vi "Measurement Logic.vi"(8 "error in":errorcluster, 9 "measurement configuration":T2 {"Baudrate" format="%x"; "FD Baudrate" format="%x"}, 10 "measure call context in":refnum<class "Measure Call Context.lvclass">, 11 "Stop OOB Server UE":refnum<user-event>) -> (0 "error out":errorcluster, 1 "measurement results":T1, 2 "measure call context out":refnum<class "Measure Call Context.lvclass">)   [LabVIEW 2025, in "CAN-LIN Raw Bus Capture.lvclass"]
doc: "Contains the core logic for executing the measurement."
uses:
  CAN-LIN Raw Bus Capture.lvclass
  <vilib>/Plug-In SDKs/Measurements/Measure Call Context/Measure Call Context.lvclass
  Measurement Configuration.ctl
  CAN-LIN Raw Bus Capture UI/Toggle.ctl
  Measurement Results.ctl
  <vilib>/xnet/xnet.llb/XNET Read (State LIN Comm).vi
  CAN-LIN Raw Bus Capture.lvclass/CAN-LIN Raw Bus Capture.ctl
  <vilib>/xnet/xnet.llb/XNET Read (State CAN Comm).vi
  <vilib>/xnet/xnet.llb/XNET Read (Frame CAN).vi
  <vilib>/xnet/xnet.llb/XNET Read (Frame LIN).vi
  OOB Data Transfer/OOB Data Transfer.lvlib
  session-management/xnetCAN/Session Management xnetCAN.lvlib
  <vilib>/Plug-In SDKs/Clients/Session Management V1/Session Reservation/Session Reservation.lvclass
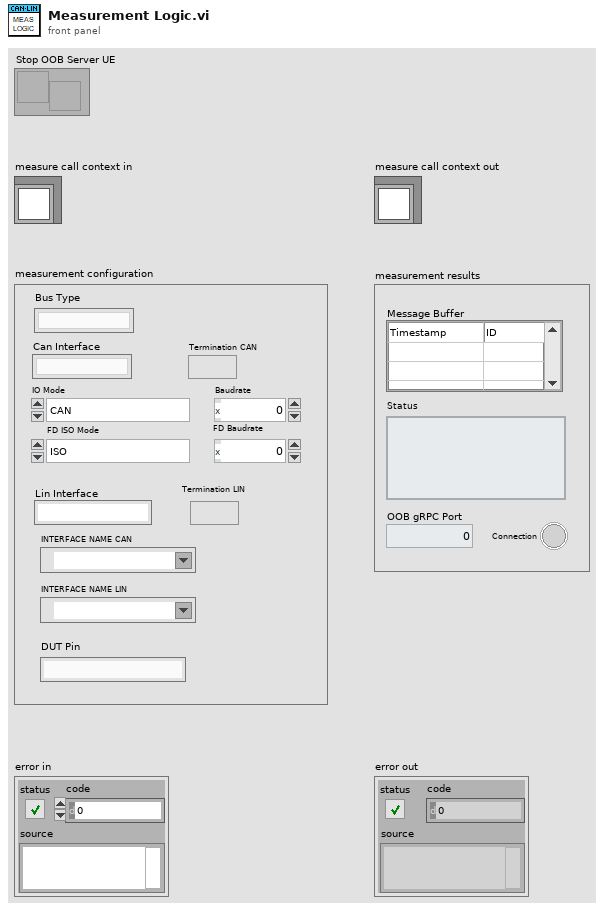
[diagram p1: front panel]
types:
  T1 = typedef "CAN-LIN Raw Bus Capture.lvclass/Measurement Results.ctl" = cluster{"Message Buffer":string[][], "Status":string, "OOB gRPC Port":i32, "Connection":bool}
  T2 = typedef "CAN-LIN Raw Bus Capture.lvclass/Measurement Configuration.ctl" = cluster{"Termination CAN":T3, "FD Baudrate":u32, "Baudrate":u32, "FD ISO Mode":enum32{"ISO", "Legacy ISO", "Non-ISO"}, "IO Mode":enum32{"CAN", "CAN FD", "CAN FD + BRS"}, "Termination LIN":T3, "Can Interface":string, "Lin Interface":string, "Bus Type":string, "INTERFACE NAME CAN":refnum<k21>, "INTERFACE NAME LIN":refnum<k21>, "DUT Pin":string}
  T3 = typedef "Toggle.ctl" = bool
  T4 = typedef "Session Management xnetCAN.lvlib/Connection with Session.ctl" = cluster{"connection":T5, "session":string}
  T5 = typedef "NI Session Management V1 Client.lvlib/Session Reservation.lvclass/Connection.ctl" = cluster{"pin or relay name":string, "site":i32, "instrument type id":string, "channel":string}
  T6 = typedef "OOB Data Transfer.lvlib/OOB to Logic Data.ctl" = cluster{"PauseResume":bool, "Export":string, "STOP":bool}
  T7 = typedef "XNET Frame CAN.ctl" = cluster{"timestamp":timestamp, "payload":u8[], "identifier":u32, "type":T8, "extended?":bool, "echo?":bool}
  T8 = typedef "XNET Frame Type CAN.ctl" = u8
  T9 = typedef "XNET CAN Comm.ctl" = cluster{"fault code":i32, "fault?":bool, "communication state":T10, "last error":T11, "receive error counter":u8, "transmit error counter":u8, "transceiver error?":bool, "sleep?":bool}
  T10 = typedef "XNET CAN Comm State.ctl" = u8
  T11 = typedef "XNET CAN Last Err.ctl" = u8
  T12 = typedef "XNET Frame LIN.ctl" = cluster{"timestamp":timestamp, "payload":u8[], "identifier":u32, "type":T13, "event ID":u8, "event slot?":bool, "echo?":bool}
  T13 = typedef "XNET Frame Type LIN.ctl" = u8
  T14 = typedef "XNET LIN Comm.ctl" = cluster{"fault code":i32, "fault?":bool, "communication state":T15, "last error":T16, "last error received":u8, "last error expected":u8, "last error identifier":u8, "sleep?":bool, "transceiver ready?":bool, "schedule index":u8}
  T15 = typedef "XNET LIN Comm State.ctl" = u8
  T16 = typedef "XNET LIN Last Err.ctl" = u8
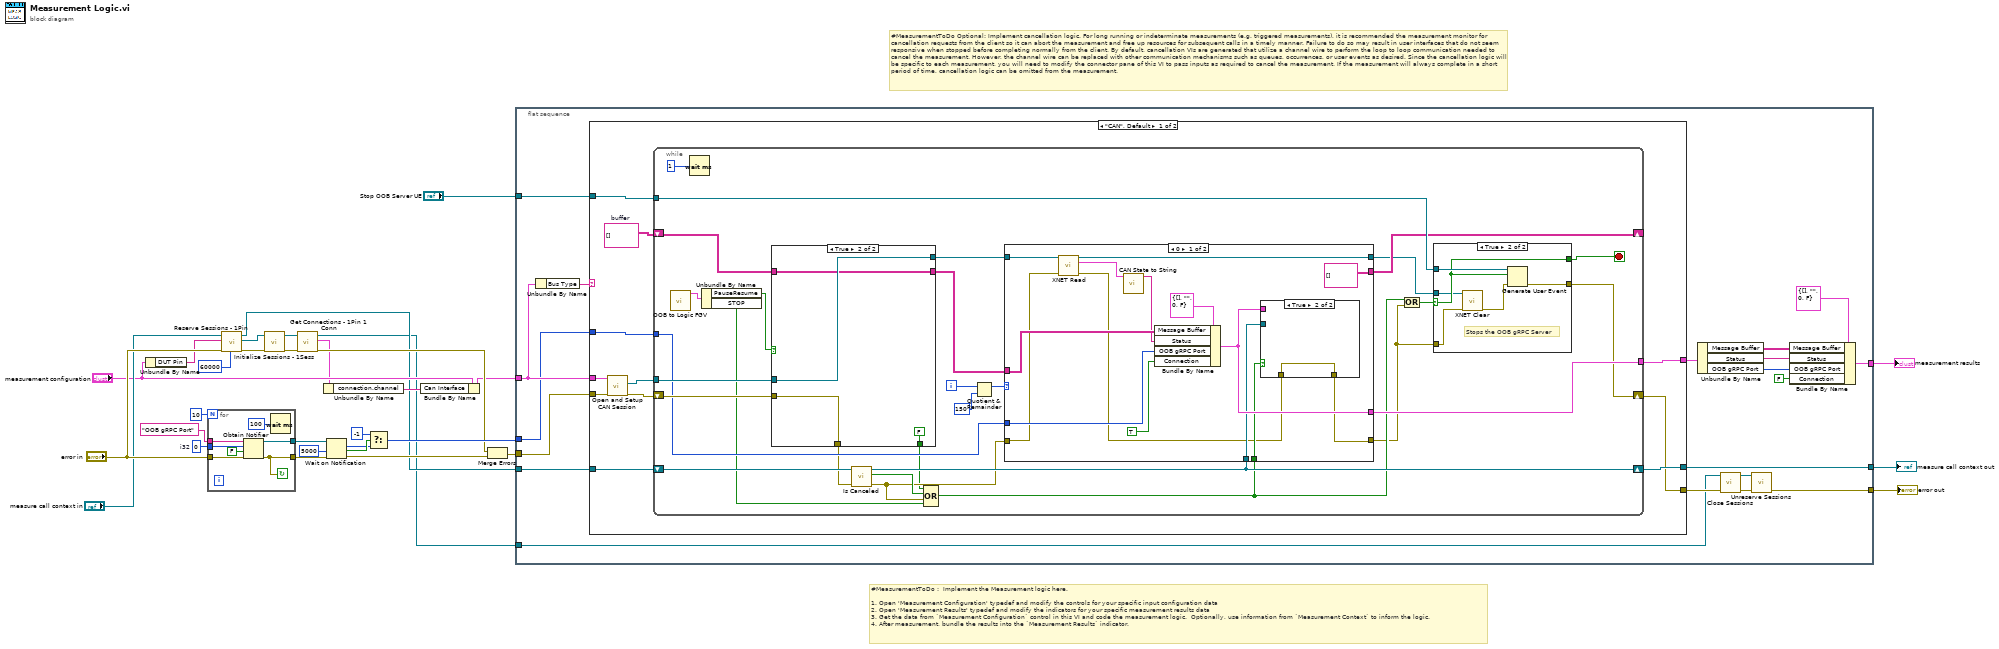
[diagram p0: block diagram]
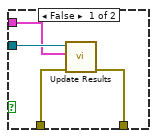
[diagram p2: hidden frame]
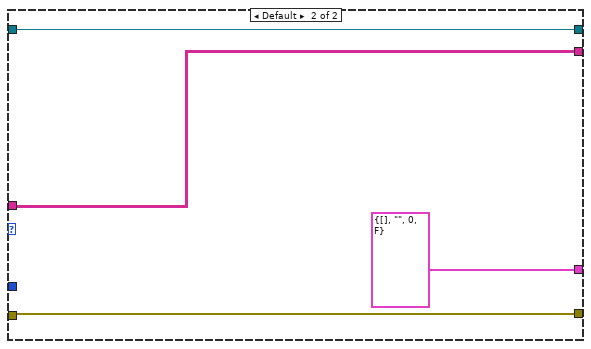
[diagram p3: hidden frame]
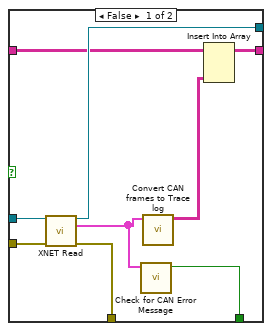
[diagram p4: hidden frame]
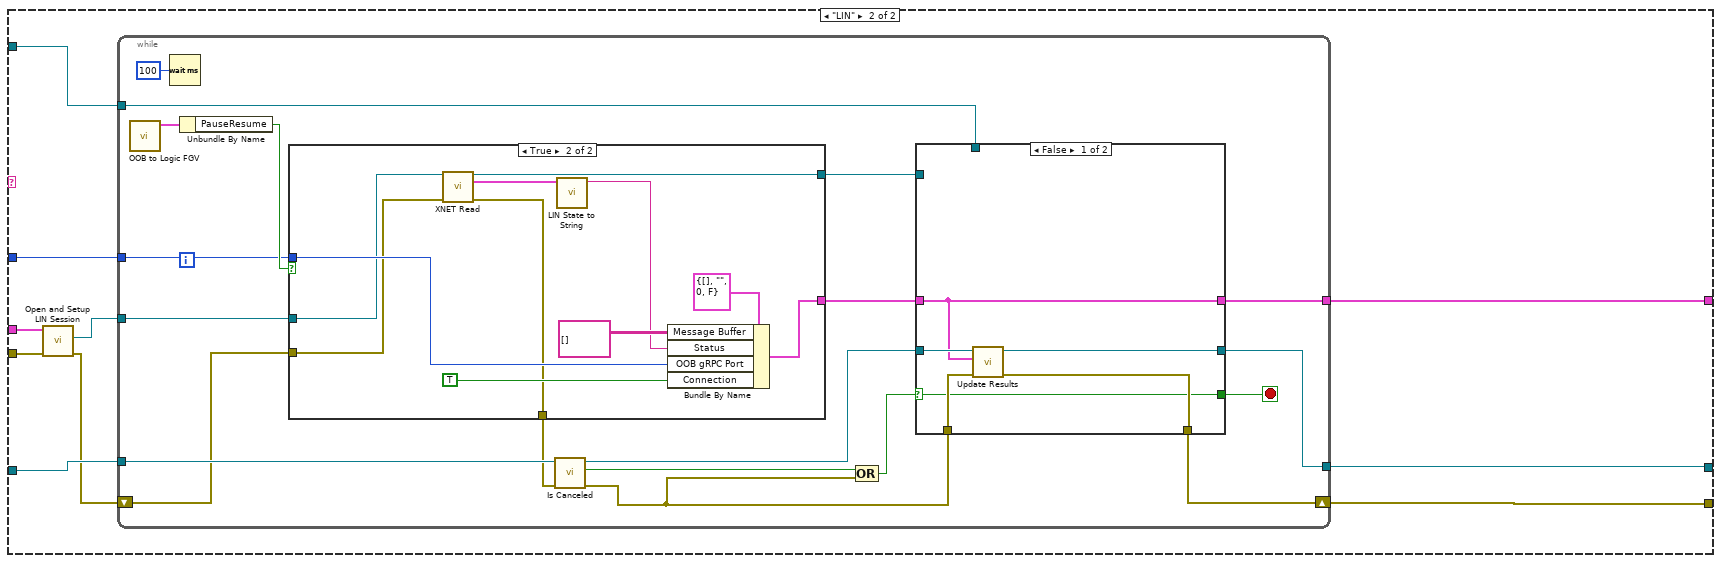
[diagram p6: hidden frame]
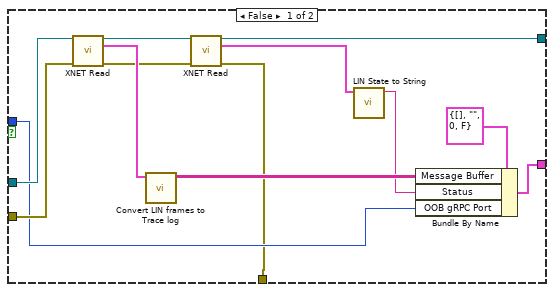
[diagram p7: hidden frame]
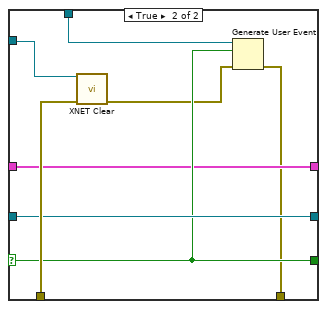
[diagram p8: hidden frame]
diagram:
  w23 = 0  # i32
  # "#MeasurementToDo Optional: Implement cancellation logic. For long running or indeterminate measurements (e.g. triggered measurements), it is recommended the measurement monitor for cancellation requests from the client so it can abort the measurement and free up resources for subsequent calls in a timely manner. Failure to do so may result in user interfaces that do not seem responsive when stopped before completing normally from the client. By default, cancellation VIs are generated that utilize a channel wire to perform the loop to loop communication needed to cancel the measurement. However, the channel wire can be replaced with other communication mechanisms such as queues, occurrences, or user events as desired. Since the cancellation logic will be specific to each measurement, you will need to modify the connector pane of this VI to pass inputs as required to cancel the measurement. If the measurement will always complete in a short period of time, cancellation logic can be omitted from the measurement."
  # "#MeasurementToDo :  Implement the Measurement logic here.\n\n1. Open 'Measurement Configuration' typedef and modify the controls for your specific input configuration data\n2. Open 'Measurement Results' typedef and modify the indicators for your specific measurement results data\n3. Get the data from `Measurement Configuration` control in this VI and code the measurement logic.  Optionally, use information from `Measurement Context` to inform the logic.\n4. After measurement, bundle the results into the `Measurement Results` indicator."
  n1 = Unbundle By Name("measurement configuration") -> ("DUT Pin"=w6:string)
  n2 = for {
    N: 10 -> [_]
    tunnel: [w35] -> w27
    tunnel: [w37] -> w26
    tunnel: "OOB gRPC Port" ("name (unnamed)") -> [w34]
    tunnel: w23 -> [w33]
    tunnel: "error in" -> [w32]
    stop <- w35 continue-if-true
    n3 = Obtain Notifier(name (unnamed)=w34, notification data type=w33, create if not found? (T)=FALSE, error in (no error)=w32) -> (notifier out=w37:refnum<notifier>, error out=w35:errorcluster)  [unwired: 1 out]
    n4 = Wait (ms)(milliseconds to wait=u32 100) -> ()  [unwired: 1 out]
  }
  n5 = call <vilib>:"Reserve Sessions - 1Pin.vi"("timeout (ms)"=60000 ("timeout in milliseconds"), "error in"="error in", "pin or relay name"=w6, "measurement context in"="measure call context in") -> ("error out"=w14:errorcluster, "session reservation out"=w15:refnum<class "Session Reservation.lvclass">, "measurement context out"=w2:refnum<class "Measure Call Context.lvclass">)  [unwired: 5 in]
  n6 = call "Initialize Sessions - 1Sess.vi"("error in"=w14, "session reservation in"=w15) -> ("error out"=w12:errorcluster, "session reservation out"=w13:refnum<class "Session Reservation.lvclass">)  [unwired: 6 in, 2 out]
  n7 = call "Get Connections - 1Pin 1 Conn.vi"("error in"=w12, "session reservation in"=w13) -> ("error out"=w9:errorcluster, "connection"=w4:T4, "session reservation out"=w1:refnum<class "Session Reservation.lvclass">)  [unwired: 7 in]
  n8 = Unbundle By Name(w4) -> ("connection.channel"=w3:string)
  n9 = Wait on Notification(notifier=w26, timeout in ms (-1)=5000, error in (no error)=w27) -> (notification=w20:i32, timed out?=w21:bool, error out=w18:errorcluster)  [unwired: 1 in, 1 out]
  n10 = Select(t=-1, s=w21, f=w20) -> (s? t:f=w17:i32)
  n11 = Bundle By Name(cluster="measurement configuration", "Can Interface"=w3) -> (w5:T2)
  n12 = Merge Errors(w9, w18) -> (w10:errorcluster)
  n13 = flat-sequence {
    tunnel: w5 -> [w56]
    tunnel: [w49] -> w31
    tunnel: w10 -> [w54]
    tunnel: w2 -> [w55]
    tunnel: [w41] -> w30
    tunnel: [w53] -> w29
    tunnel: "Stop OOB Server UE" -> [w52]
    tunnel: w17 -> [w51]
    tunnel: w1 -> [w40]
    frame #0 {
      n14 = Unbundle By Name(w56) -> ("Bus Type"=w57:string)
      n15 = case shown="\"CAN\", Default" w57 {
        tunnel: w56 -> [w66 w145]
        tunnel: w55 -> [w65 w148]
        tunnel: w54 -> [w64 w147]
        tunnel: [w63 w149] -> w50
        tunnel: [w62 w151] -> w53
        tunnel: [w61 w150] -> w42
        tunnel: w52 -> [w60 w143]
        tunnel: w51 -> [w59 w142]
        frame "CAN", Default {
          w58 = string[][] []  # buffer
          n16 = call "Open and Setup CAN Session.vi"("error in"=w64, "measurement configuration"=w66) -> ("error out"=w67:errorcluster, "session out"=w68:refnum<k21>)  [unwired: 8 in]
          n17 = while {
            tunnel: [w87] -> w63
            shift-right: [w76] -> w61
            shift-left: w67 -> [w94]
            tunnel: w68 -> [w93]
            tunnel: w60 -> [w92]
            tunnel: w59 -> [w89]
            shift-right: [w81] -> w62
            shift-left: w65 -> [w95]
            shift-right: [w78] -> _
            shift-left: w58 -> [w83]
            i -> [w86]
            stop <- w70 stop-if-true
            n18 = call "OOB to Logic FGV.vi"() -> ("OOB to Logic Data out"=w90:T6)  [unwired: 10 in, 1 out]
            n19 = Wait (ms)(milliseconds to wait=u32 1) -> ()  [unwired: 1 out]
            n20 = Unbundle By Name(w90) -> ("PauseResume"=w77:bool, "STOP"=w69:bool)
            n21 = case shown="True" w77 {
              tunnel: w94 -> [w129 w133]
              tunnel: [w128 w133] -> w88
              tunnel: [w127 w132] -> w79
              tunnel: w93 -> [w126 w132]
              tunnel: w83 -> [w125 w131]
              tunnel: [w123 w131] -> w82
              tunnel: [w121 FALSE ("Error")] -> w71
              frame False {
                n22 = call-poly <vilib>:"XNET Read.vi"("session in"=w126, "error in (no error)"=w129) -> ("session out"=w127:refnum<k21>, "data"=w122:T7[], "error out"=w128:errorcluster)  [unwired: 10 in, 1 out]
                n23 = call "Check for CAN Error Message.vi"("data"=w122) -> ("Error"=w121:bool)  [unwired: 9 in, 1 out]
                n24 = call "Convert CAN frames to Trace log.vi"("can frames in"=w122) -> ("trace out"=w124:string[][])  [unwired: 10 in]
                n25 = Insert Into Array(array=w125, new element=w124) -> (w123:string[][])  [unwired: 2 in]
              }
              frame True {
              }
            }
            n26 = call <vilib>:"Is Canceled.vi"("error in"=w88, "measure call context in"=w95) -> ("error out"=w80:errorcluster, "is canceled?"=w91:bool, "measure call context out"=w81:refnum<class "Measure Call Context.lvclass">)  [unwired: 7 in]
            n27 = Compound Arithmetic op=OR(w71, w91, w80, w69) -> (w74:bool)
            n28 = Quotient & Remainder(x=w86, y=150) -> (x-y*floor(x/y)=w84:i32)  [unwired: 1 out]
            n29 = case shown="0" w84 {
              tunnel: w89 -> [w110 _]
              tunnel: [w109 T1 {"Message Buffer"=[], "Status"="", "OOB gRPC Port"=0, "Connection"=FALSE} ("Measurement Results")] -> w87
              tunnel: w82 -> [w104 w119]
              tunnel: w74 -> [w108 _]
              tunnel: w81 -> [w107 _]
              tunnel: w80 -> [w102 w120]
              tunnel: w79 -> [w103 w117]
              tunnel: [w106 w120] -> w73
              tunnel: [string[][] [] ("buffer") w119] -> w78
              tunnel: [w97 w117] -> w75
              frame 0 {
                n30 = call-poly <vilib>:"XNET Read.vi"("session in"=w103, "error in (no error)"=w102) -> ("session out"=w97:refnum<k21>, "CAN comm"=w100:T9, "error out"=w101:errorcluster)  [unwired: 11 in]
                n31 = call "CAN State to String.vi"("CAN comm in"=w100) -> ("string out"=w99:string)  [unwired: 10 in]
                n32 = Bundle By Name(cluster=T1 {"Message Buffer"=[], "Status"="", "OOB gRPC Port"=0, "Connection"=FALSE} ("Measurement Results"), "Message Buffer"=w104, "Status"=w99, "OOB gRPC Port"=w110, "Connection"=TRUE) -> (w109:T1)
                n33 = case shown="True" w108 {
                  tunnel: w107 -> [w115 _]
                  tunnel: w101 -> [w114 w116]
                  tunnel: [w113 w116] -> w106
                  tunnel: w109 -> [w112 _]
                  frame False {
                    n34 = call <vilib>:"Update Results.vi"("error in"=w114, "measurement results"=w112, "measure call context in"=w115) -> ("error out"=w113:errorcluster)  [unwired: 7 in, 1 out]
                  }
                  frame True {
                  }
                }
              }
              frame Default {
              }
            }
            n35 = Compound Arithmetic op=OR(w74, w73) -> (w72:bool)
            n36 = case shown="True" w72 {
              selector: w72 -> [w135 w140]
              tunnel: w92 -> [_ w141]
              tunnel: [w135 w140] -> w70
              tunnel: w73 -> [w134 w137]
              tunnel: [w134 w139] -> w76
              tunnel: w75 -> [_ w138]
              frame False {
              }
              frame True {
                # "Stops the OOB gRPC Server"
                n37 = call <vilib>:"XNET Clear.vi"("session in"=w138, "error in (no error)"=w137) -> ("error out"=w136:errorcluster)  [unwired: 13 in]
                n38 = Generate User Event(user event=w141, event data cluster=w140, error in=w136) -> (error out=w139:errorcluster)  [unwired: 1 in, 1 out]
              }
            }
          }
        }
        frame "LIN" {
          n39 = call "Open and Setup LIN Session.vi"("error in"=w147, "measurement configuration"=w145) -> ("error out"=w146:errorcluster, "session out"=w144:refnum<k21>)  [unwired: 8 in]
          n40 = while {
            tunnel: [w152] -> w149
            tunnel: w148 -> [w169]
            tunnel: [w166] -> w151
            shift-right: [w160] -> w150
            shift-left: w146 -> [w168]
            tunnel: w144 -> [w163]
            tunnel: w143 -> [w154]
            tunnel: w142 -> [w156]
            stop <- w153 stop-if-true
            n41 = call "OOB to Logic FGV.vi"() -> ("OOB to Logic Data out"=w162:T6)  [unwired: 10 in, 1 out]
            n42 = Wait (ms)(milliseconds to wait=u32 100) -> ()  [unwired: 1 out]
            n43 = Unbundle By Name(w162) -> ("PauseResume"=w161:bool)
            n44 = case shown="True" w161 {
              tunnel: w168 -> [w182 w185]
              tunnel: [w171 w184] -> w155
              tunnel: [w175 w189] -> w165
              tunnel: [w181 w192] -> w164
              tunnel: w163 -> [w180 w190]
              tunnel: w156 -> [w177 w191]
              frame False {
                n45 = call-poly <vilib>:"XNET Read.vi"("session in"=w180, "error in (no error)"=w182) -> ("session out"=w176:refnum<k21>, "data"=w179:T12[], "error out"=w172:errorcluster)  [unwired: 10 in, 1 out]
                n46 = call "Convert LIN frames to Trace log.vi"("lin frames in"=w179) -> ("trace out"=w178:string[][])  [unwired: 10 in]
                n47 = call-poly <vilib>:"XNET Read.vi"("session in"=w176, "error in (no error)"=w172) -> ("session out"=w175:refnum<k21>, "LIN comm"=w174:T14, "error out"=w171:errorcluster)  [unwired: 11 in]
                n48 = call "LIN State to String.vi"("LIN comm in"=w174) -> ("string out"=w173:string)  [unwired: 10 in]
                n49 = Bundle By Name(cluster=T1 {"Message Buffer"=[], "Status"="", "OOB gRPC Port"=0, "Connection"=FALSE} ("Measurement Results"), "Message Buffer"=w178, "Status"=w173, "OOB gRPC Port"=w177) -> (w181:T1)
              }
              frame True {
                n50 = call-poly <vilib>:"XNET Read.vi"("session in"=w190, "error in (no error)"=w185) -> ("session out"=w189:refnum<k21>, "LIN comm"=w188:T14, "error out"=w184:errorcluster)  [unwired: 11 in]
                n51 = call "LIN State to String.vi"("LIN comm in"=w188) -> ("string out"=w187:string)  [unwired: 10 in]
                n52 = Bundle By Name(cluster=T1 {"Message Buffer"=[], "Status"="", "OOB gRPC Port"=0, "Connection"=FALSE} ("Measurement Results"), "Message Buffer"=string[][] [], "Status"=w187, "OOB gRPC Port"=w191, "Connection"=TRUE) -> (w192:T1)
              }
            }
            n53 = call <vilib>:"Is Canceled.vi"("error in"=w155, "measure call context in"=w169) -> ("error out"=w159:errorcluster, "is canceled?"=w158:bool, "measure call context out"=w167:refnum<class "Measure Call Context.lvclass">)  [unwired: 7 in]
            n54 = Compound Arithmetic op=OR(w158, w159) -> (w157:bool)
            n55 = case shown="False" w157 {
              selector: w157 -> [w196 w204]
              tunnel: w167 -> [w200 w206]
              tunnel: w159 -> [w199 w208]
              tunnel: [w198 w201] -> w160
              tunnel: [w197 w206] -> w166
              tunnel: w165 -> [_ w207]
              tunnel: w164 -> [w195 w203]
              tunnel: w154 -> [_ w205]
              tunnel: [w196 w204] -> w153
              tunnel: [w195 w203] -> w152
              frame False {
                n56 = call <vilib>:"Update Results.vi"("error in"=w199, "measurement results"=w195, "measure call context in"=w200) -> ("error out"=w198:errorcluster, "measure call context out"=w197:refnum<class "Measure Call Context.lvclass">)  [unwired: 7 in]
              }
              frame True {
                n57 = call <vilib>:"XNET Clear.vi"("session in"=w207, "error in (no error)"=w208) -> ("error out"=w202:errorcluster)  [unwired: 13 in]
                n58 = Generate User Event(user event=w205, event data cluster=w204, error in=w202) -> (error out=w201:errorcluster)  [unwired: 1 in, 1 out]
              }
            }
          }
        }
      }
      n59 = Unbundle By Name(w50) -> ("Message Buffer"=w47:string[][], "Status"=w46:string, "OOB gRPC Port"=w44:i32)
      n60 = call <vilib>:"Close Sessions.vi"("error in"=w42, "session reservation in"=w40) -> ("error out"=w43:errorcluster, "session reservation out"=w39:refnum<class "Session Reservation.lvclass">)  [unwired: 8 in]
      n61 = call <vilib>:"Unreserve Sessions.vi"("error in"=w43, "session reservation in"=w39) -> ("error out"=w41:errorcluster)  [unwired: 9 in]
      n62 = Bundle By Name(cluster=T1 {"Message Buffer"=[], "Status"="", "OOB gRPC Port"=0, "Connection"=FALSE} ("Measurement Results"), "Message Buffer"=w47, "Status"=w46, "OOB gRPC Port"=w44, "Connection"=FALSE) -> (w49:T1)
    }
  }
  "error out" <- w30
  "measure call context out" <- w29
  "measurement results" <- w31
